vi "Generate Stop Event.vi"(8 "error in (no error)":errorcluster, 11 "Controller in":refnum<class "Controller.lvclass">) -> (0 "error out":errorcluster, 3 "Controller out":refnum<class "Controller.lvclass">)   [LabVIEW 2020, in "Controller.lvlib" / "Controller.lvclass"]
uses:
  Controller.lvclass
  Controller.lvclass/Controller.ctl
  Properties/Read E-Stop.vi
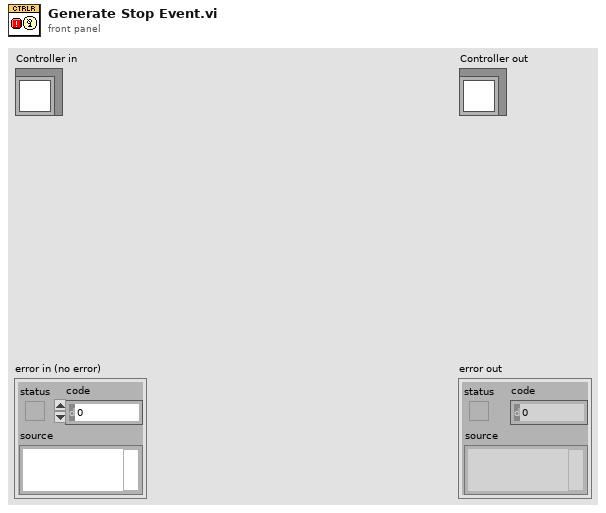
[diagram p1: front panel]
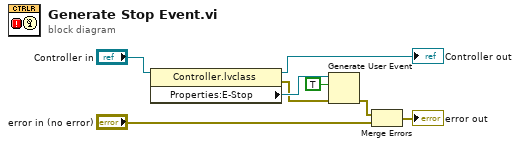
[diagram p0: block diagram]
diagram:
  n1 = property class="Controller.lvclass"(reference="Controller in") -> (reference out=→"Controller out":refnum<class "Controller.lvclass">, error out=w4:errorcluster, "Properties:E-Stop"=w5:refnum<user-event>)  [unwired: 1 in]
  n2 = Generate User Event(user event=w5, event data cluster=TRUE ("event data"), error in=w4) -> (error out=w3:errorcluster)  [unwired: 1 in, 1 out]
  n3 = Merge Errors(w3, "error in (no error)") -> (→"error out":errorcluster)
